vi "commTest.vi"() -> ()   [LabVIEW 2012]
panel:
  out "cmd out":T1
  in  "停止 2":bool
  out "数值 2":i32
  out "错误输出":errorcluster
  out "data out":string
  out "数值":i32
  out "error out":errorcluster caption="错误输出"
  out "remote address":string caption="远程地址"
  out "remote port":u16 caption="远程端口"
  in  "停止":bool
  out "out":string
  in  "in":string
  in  "布尔":bool
  in  "Msg":T2
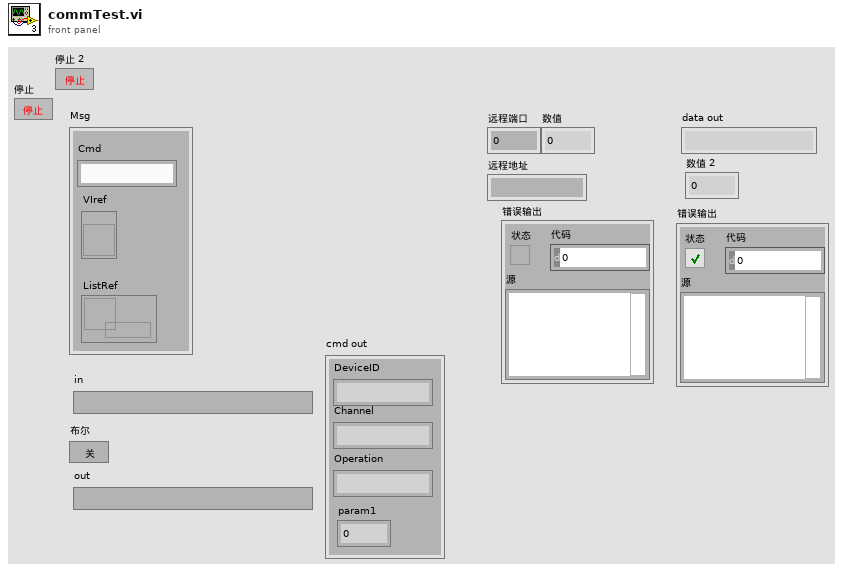
[diagram p1: front panel]
types:
  T1 = cluster{"DeviceID":string, "Channel":string, "param1":dbl, "Operation":string}
  T2 = cluster{"Cmd":string, "VIref":refnum<vi>, "ListRef":refnum<queue>}
  T3 = enum16{"Standard", "Buffered", "CRLF", "Immediate"}
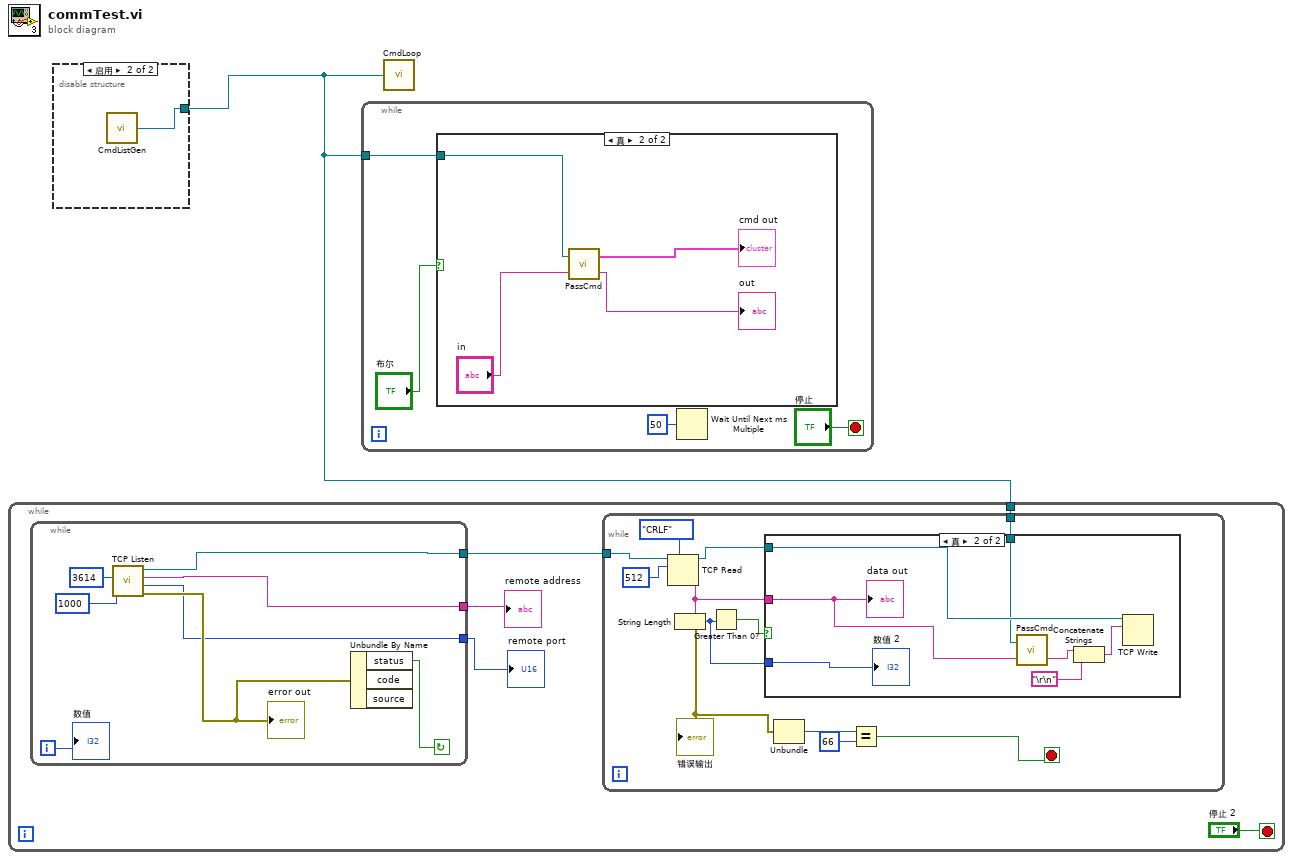
[diagram p0: block diagram]
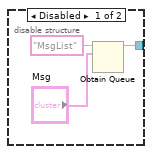
[diagram p2: hidden frame]
diagram:
  n1 = disable-structure shown="启用" {
    disable-tunnel: [w2 w5] -> w1
    frame Disabled {
      n2 = Obtain Queue(name (unnamed)="MsgList" ("名称（未命名）"), element data type="Msg") -> (queue out=w2:refnum<queue>)  [unwired: 3 in, 2 out]
    }
    frame Enabled {
      n3 = call "CmdListGen.vi"() -> ("队列输出"=w5:refnum<queue>)  [unwired: 1 in]
    }
  }
  n4 = while {
    tunnel: w1 -> [w7]
    stop <- "停止 2" stop-if-true
    n5 = while {
      tunnel: [w35] -> w8
      tunnel: [w32] -> w10
      tunnel: [w31] -> w9
      i -> [w30]
      stop <- w33 continue-if-true
      n6 = call <vilib>:"TCP Listen.vi"("timeout ms (wait forever: -1)"=1000, "port"=u16 3614) -> ("error out"=w34:errorcluster, "remote port"=w31:u16, "remote address"=w32:string, "connection ID"=w35:refnum<k5>)  [unwired: 5 in, 1 out]
      "error out" <- w34
      n7 = Unbundle By Name(w34) -> ("status"=w33:bool)  [unwired: 2 out]
      "数值" <- w30
    }
    "remote address" <- w10
    "remote port" <- w9
    n8 = while {
      tunnel: w8 -> [w13]
      tunnel: w7 -> [w11]
      stop <- w15 stop-if-true
      n9 = TCP Read(connection ID=w13, bytes to read=512 ("读取的字节"), 7:T3."CRLF" ("模式（标准）")) -> (connection ID out=w12:refnum<k5>, data out=w19:string, error out=w18:errorcluster)  [unwired: 2 in]
      "错误输出" <- w18
      n10 = String Length(string=w19) -> (length=w14:i32)
      n11 = Greater Than 0?(x=w14) -> (x > 0?=w20:bool)
      n12 = case shown="真" w20 {
        tunnel: w19 -> [_ w27]
        tunnel: w14 -> [_ w29]
        tunnel: w12 -> [_ w28]
        tunnel: w11 -> [_ w26]
        frame False {
        }
        frame True {
          n13 = call "PassCmd.vi"("cmd in"=w27, "list ref"=w26) -> ("str out"=w25:string)  [unwired: 1 out]
          n14 = Concatenate Strings(w25, "\r\n") -> (w24:string)
          n15 = TCP Write(connection ID=w28, data in=w24) -> ()  [unwired: 2 in, 3 out]
          "data out" <- w27
          "数值 2" <- w29
        }
      }
      n16 = Unbundle(w18) -> ("code"=w17:i32)  [unwired: 2 out]
      n17 = Equal?(x=w17, y=66) -> (x = y?=w15:bool)
    }
  }
  n18 = while {
    tunnel: w1 -> [w40]
    stop <- "停止" stop-if-true
    n19 = case shown="真" "布尔" {
      tunnel: w40 -> [_ w42]
      frame False {
      }
      frame True {
        n20 = call "PassCmd.vi"("cmd in"="in", "list ref"=w42) -> ("str out"=→"out":string, "cmd out"=→"cmd out":T1)
      }
    }
    n21 = Wait Until Next ms Multiple(millisecond multiple=u32 50 ("毫秒倍数")) -> ()  [unwired: 1 out]
  }
  n22 = call "CmdLoop.vi"("ListRef"=w1) -> ()  [unwired: 1 out]
